vi "globalVar.vi"(6 "action":T1=enum."Set", 11 "Param in":T2) -> (3 "Param in 2":T2)   [LabVIEW 2019]
uses:
  paramIn.ctl
  action.ctl
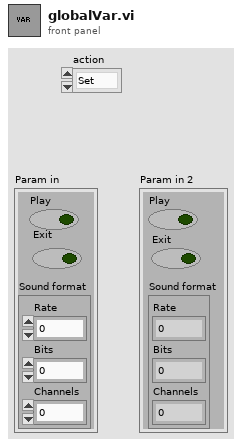
[diagram p1: front panel]
types:
  T1 = typedef "action.ctl" = enum16{"Get", "Set"}
  T2 = typedef "paramIn.ctl" = cluster{"Play":bool, "Sound format":cluster{"Rate":i32, "Bits":i32, "Channels":u32}, "Exit":bool}
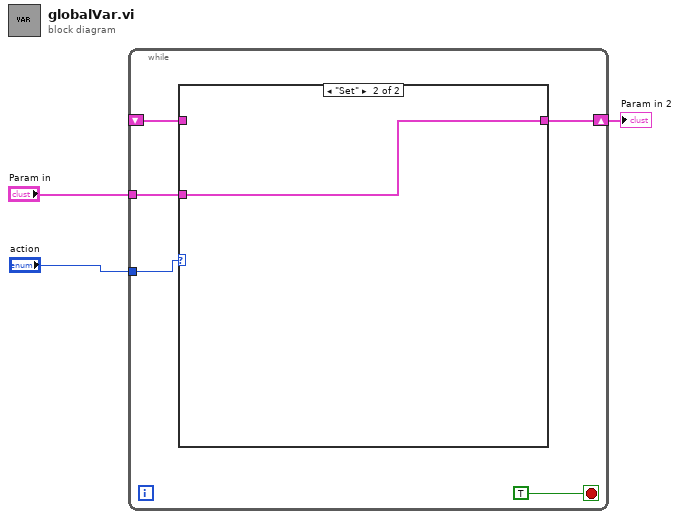
[diagram p0: block diagram]
diagram:
  n1 = while {
    tunnel: "action" -> [w8]
    tunnel: "Param in" -> [w6]
    shift-right: [w5] -> w2
    shift-left: _ -> [w4]
    stop <- TRUE stop-if-true
    n2 = case shown="\"Set\"" w8 {
      tunnel: w6 -> [_ w10]
      tunnel: [w9 w10] -> w5
      tunnel: w4 -> [w9 _]
      frame "Get", Default {
      }
      frame "Set" {
      }
    }
  }
  "Param in 2" <- w2
